vi "(Depricated) Sample In Transfer Line.vi"(8 "error in (no error)":errorcluster, 10 "Sample In":refnum<class "Sample.lvclass">, 11 "cRIO-CO2 in":refnum<class "cRIO-CO2.lvclass">=refnum) -> (0 "error out":errorcluster, 3 "cRIO-CO2 out":refnum<class "cRIO-CO2.lvclass">)   [LabVIEW 2015, in "cRIO-CO2.lvclass"]
uses:
  cRIO-CO2.lvclass
  subs/Sample/Sample.lvclass
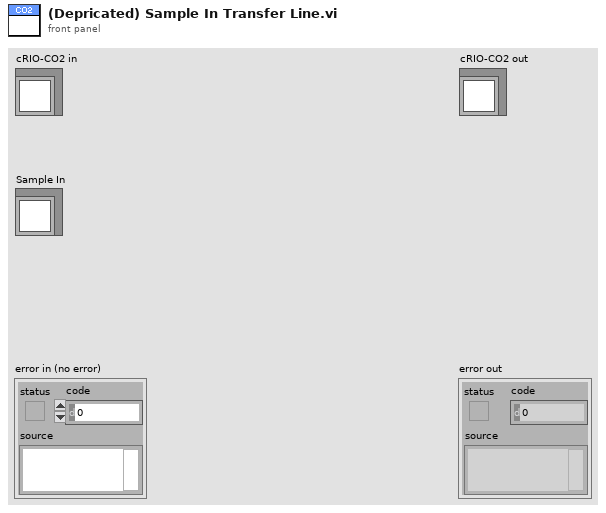
[diagram p1: front panel]
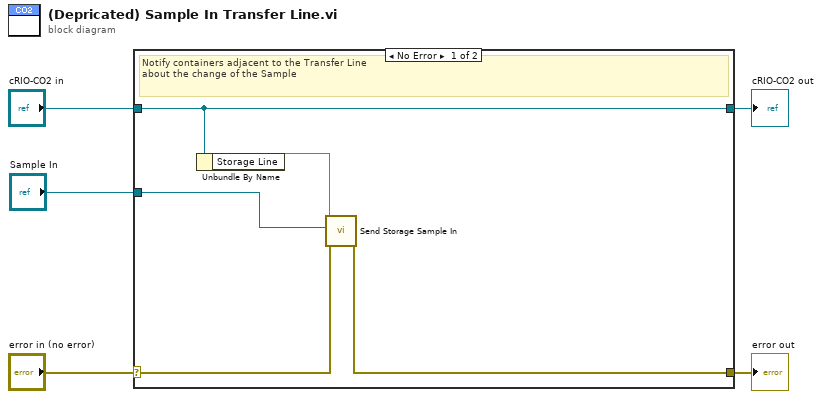
[diagram p0: block diagram]
diagram:
  n1 = case shown="No Error" "error in (no error)" {
    selector: "error in (no error)" -> [w7 w12]
    tunnel: [w6 w12] -> w4
    tunnel: [w10 w11] -> w2
    tunnel: "cRIO-CO2 in" -> [w10 w11]
    tunnel: "Sample In" -> [w8 _]
    frame No Error {
      # "Notify containers adjacent to the Transfer Line\nabout the change of the Sample"
      n2 = Unbundle By Name(w10) -> ("Storage Line"=w9)
      n3 = call "Send Storage Sample In.vi"("error in (no error)"=w7, "Sample In"=w8, "Message Enqueuer"=w9) -> ("error out"=w6:errorcluster)  [unwired: 7 in, 1 out]
    }
    frame Error {
    }
  }
  "error out" <- w4
  "cRIO-CO2 out" <- w2
